vi "Build Control Type.vi"(8 "error in (no error)":errorcluster, 11 "Control Builder in":refnum<class "GUI Control Builder.lvclass">) -> (0 "error out":errorcluster, 2 "GUI Control":refnum<class "GUI Control.lvclass">, 3 "Control Builder out":refnum<class "GUI Control Builder.lvclass">)   [LabVIEW 2015, in "GUI Control Builder.lvclass"]
uses:
  GUI Control Builder.lvclass
  GUI Controls/GUI Control/GUI Control.lvclass
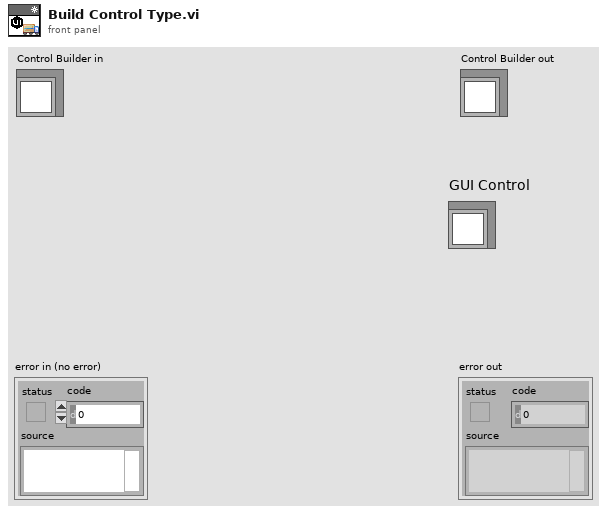
[diagram p1: front panel]
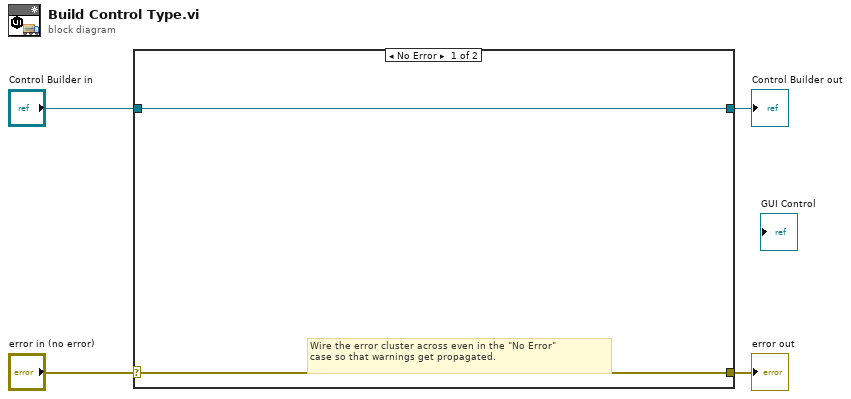
[diagram p0: block diagram]
diagram:
  n1 = case shown="No Error" "error in (no error)" {
    selector: "error in (no error)" -> [w6 w8]
    tunnel: [w6 w8] -> w3
    tunnel: [w5 w7] -> w1
    tunnel: "Control Builder in" -> [w5 w7]
    frame No Error {
      # "Wire the error cluster across even in the \"No Error\"\ncase so that warnings get propagated."
    }
    frame Error {
    }
  }
  "error out" <- w3
  "Control Builder out" <- w1
